vi "focuscamera.vi"(2 "RetPos":bool, 3 "Wait":bool=TRUE, 4 "addition":sgl, 5 "MG17Motor":refnum<k7>(container)) -> (0 "StartPosition(um)":sgl, 1 "EndPosition (um)":sgl)   [LabVIEW 2013]
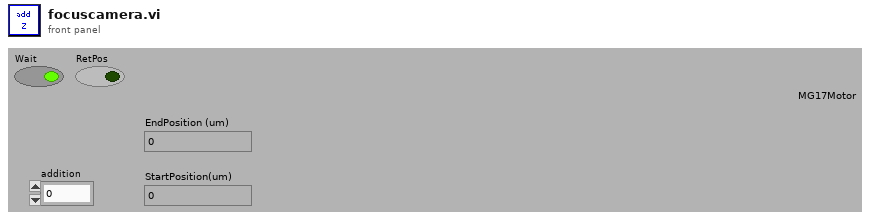
[diagram p1: front panel]
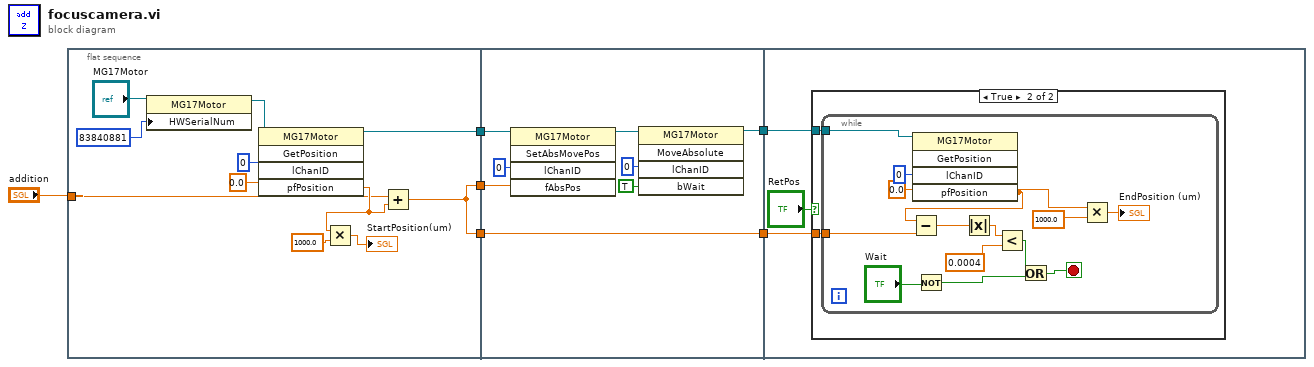
[diagram p0: block diagram]
diagram:
  n1 = flat-sequence {
    tunnel: [w16] -> w6
    tunnel: [w7] -> w5
    tunnel: "addition" -> [w8]
    tunnel: [w7] -> w1
    tunnel: w6 -> [w25]
    tunnel: w5 -> [w23]
    tunnel: [w19] -> w4
    tunnel: [w18] -> w2
    tunnel: w1 -> [w18]
    tunnel: w4 -> [w28]
    tunnel: w2 -> [w26]
    frame #0 {
      n2 = property class="MG17Motor"(reference="MG17Motor", "HWSerialNum"=83840881) -> (reference out=w10:refnum<k7>)  [unwired: 1 in, 1 out]
      n3 = invoke class="MG17Motor" method="GetPosition"(reference=w10, "lChanID"=0, "pfPosition"=sgl 0.0) -> (reference out=w16:refnum<k7>, "pfPosition"=w9:sgl)  [unwired: 2 in, 3 out]
      n4 = Multiply(x=w9, y=sgl 1000.0) -> (x*y=→"StartPosition(um)":sgl)
      n5 = Add(x=w8, y=w9) -> (x+y=w7:sgl)
    }
    frame #1 {
      n6 = invoke class="MG17Motor" method="SetAbsMovePos"(reference=w25, "lChanID"=0, "fAbsPos"=w23) -> (reference out=w24:refnum<k7>)  [unwired: 2 in, 4 out]
      n7 = invoke class="MG17Motor" method="MoveAbsolute"(reference=w24, "lChanID"=0, "bWait"=TRUE) -> (reference out=w19:refnum<k7>)  [unwired: 2 in, 4 out]
    }
    frame #2 {
      n8 = case shown="True" "RetPos" {
        tunnel: w28 -> [_ w30]
        tunnel: w26 -> [_ w29]
        frame False {
        }
        frame True {
          n9 = while {
            tunnel: w30 -> [w39]
            tunnel: w29 -> [w31]
            stop <- w32 stop-if-true
            n10 = invoke class="MG17Motor" method="GetPosition"(reference=w39, "lChanID"=0, "pfPosition"=sgl 0.0) -> ("pfPosition"=w37:sgl)  [unwired: 2 in, 4 out]
            n11 = Subtract(x=w37, y=w31) -> (x-y=w42:sgl)
            n12 = Not(x="Wait") -> (.not. x?=w34:bool)
            n13 = Absolute Value(x=w42) -> (abs(x)=w41:sgl)
            n14 = Less?(x=w41, y=0.0004) -> (x < y?=w33:bool)
            n15 = Or(x=w33, y=w34) -> (x .or. y?=w32:bool)
            n16 = Multiply(x=w37, y=sgl 1000.0) -> (x*y=→"EndPosition (um)":sgl)
          }
        }
      }
    }
  }
